vi "MTMount_getResponse_enableCamWrap.vi"(8 "error in (no error)":errorcluster, 11 "ackcmd_Ctl":T1={"cmdSeqNum"=0, "ack"=0, "error"=0, "result"="                                                                                                                                                                                                                                                                ", "host"=0, "origin"=0, "cmdtype"=0, "timeout"=0.0}) -> (0 "error out":errorcluster, 2 "function return":i32, 3 "ackcmd_Ctl out":T1={"cmdSeqNum"=0, "ack"=0, "error"=0, "result"="                                                                                                                                                                                                                                                                ", "host"=0, "origin"=0, "cmdtype"=0, "timeout"=0.0})   [LabVIEW 2018, in "SALLV_MTMount.lvlib"]
doc: "int MTMount_shm_getResponse_enableCamWrapLV(MTMount_ackcmdLV *ackcmd_Ctl);"
uses:
  SALLV_MTMount.lvlib
  DataTypes/ackcmd.ctl
  SALLV_MTMount.so
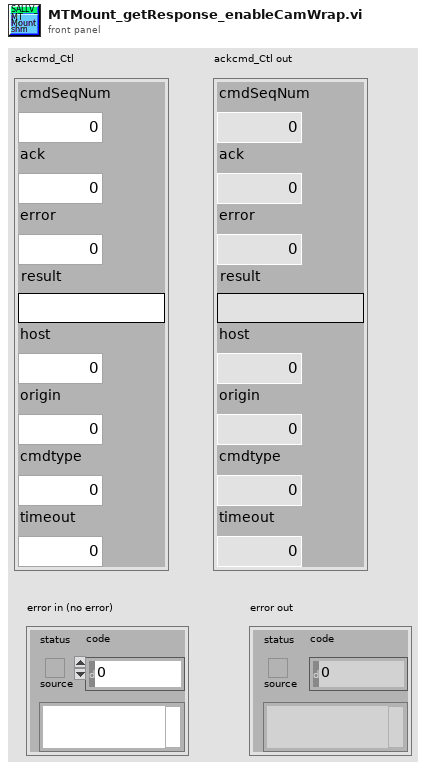
[diagram p1: front panel]
types:
  T1 = typedef "SALLV_MTMount.lvlib/ackcmd.ctl" = cluster{"cmdSeqNum":i32, "ack":i32, "error":i32, "result":string, "host":i32, "origin":i32, "cmdtype":i32, "timeout":dbl}
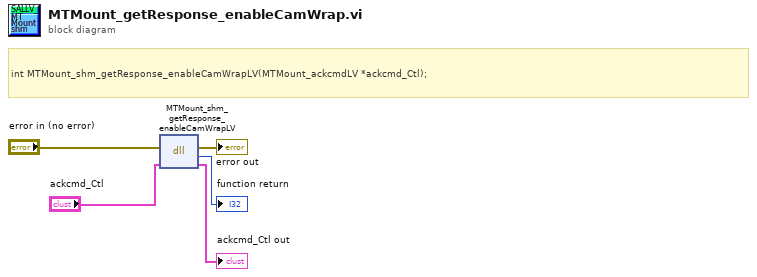
[diagram p0: block diagram]
diagram:
  # "int MTMount_shm_getResponse_enableCamWrapLV(MTMount_ackcmdLV *ackcmd_Ctl);"
  n1 = dll-call lib="home/ttsai/Document/salApiMTMount/SALLV_MTMount/SALLV_MTMount.*" fn="MTMount_shm_getResponse_enableCamWrapLV"(error in="error in (no error)", "ackcmd_Ctl"="ackcmd_Ctl") -> (error out=→"error out":errorcluster, →"function return":i32, "ackcmd_Ctl"=→"ackcmd_Ctl out":T1)  [unwired: 2 in, 1 out]
